vi "WPI_UtilitiesFRC WPILibVersion.vi"(11 "error in (no error)":errorcluster) -> (8 "Version":string, 15 "error out":errorcluster)   [LabVIEW 2019]
doc: "Returns the version of the WPI Library (WPILib) of VIs.\n\nThis software is licensed. Open the labview\\readme\\WPI Robotics Library Open Source License.txt file for more information."
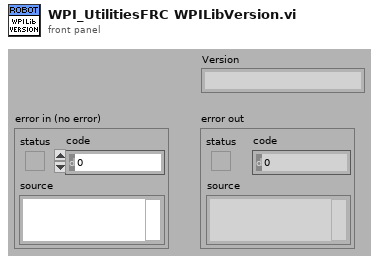
[diagram p1: front panel]
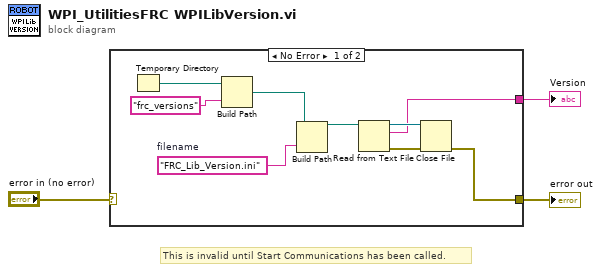
[diagram p0: block diagram]
diagram:
  # "This is invalid until Start Communications has been called."
  n1 = case shown="No Error" "error in (no error)" {
    selector: "error in (no error)" -> [_ w13]
    tunnel: [w7 w13] -> w2
    tunnel: [w9 _] -> w1
    frame No Error {
      w12 = "FRC_Lib_Version.ini"  # filename
      n2 = Temporary Directory() -> (w5:path)
      n3 = Build Path(base path=w5, name or relative path="frc_versions") -> (appended path=w4:path)
      n4 = Build Path(base path=w4, name or relative path=w12) -> (appended path=w11:path)
      n5 = Read from Text File(file (use dialog)=w11) -> (refnum out=w10:refnum<file>, text=w9:string, error out=w8:errorcluster)  [unwired: 3 in, 1 out]
      n6 = Close File(refnum=w10, error in=w8) -> (error out=w7:errorcluster)  [unwired: 1 out]
    }
    frame Error {
    }
  }
  "error out" <- w2
  "Version" <- w1
